vi "LSX Get Trigger Par.vi"(0 "lLSID":i32, 1 "pdDistance":dbl, 5 "plAxis":i32, 7 "plMode":i32, 9 "plSignal":i32, 11 "error in (no error)":errorcluster) -> (3 "pdDistance out":dbl, 4 "function return":i32, 6 "plAxis out":i32, 8 "plMode out":i32, 10 "plSignal out":i32, 15 "error out":errorcluster)   [LabVIEW 2018, in "Tango.lvlib"]
doc: "TANGOAPI int TANGOCALL LSX_GetTriggerPar (int lLSID, int *plAxis, int *plMode, int *plSignal, double *pdDistance);"
uses:
  Tango.lvlib
  SubVIs/Tango_DLL.dll
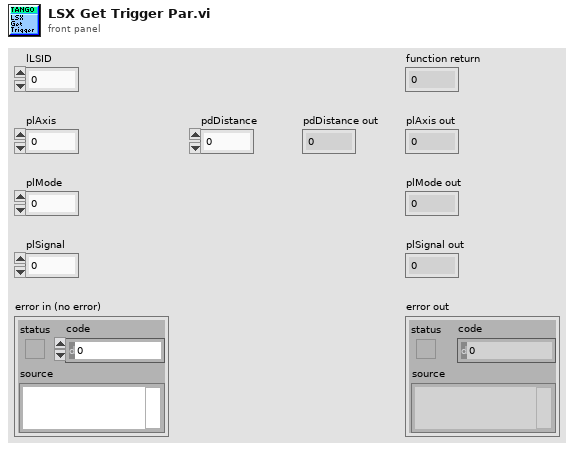
[diagram p1: front panel]
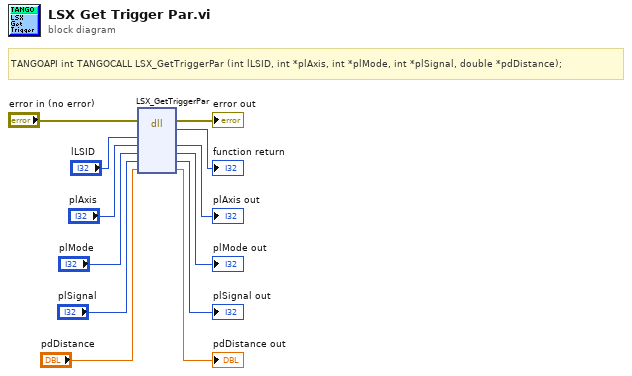
[diagram p0: block diagram]
diagram:
  # "TANGOAPI int TANGOCALL LSX_GetTriggerPar (int lLSID, int *plAxis, int *plMode, int *plSignal, double *pdDistance);"
  n1 = dll-call lib="C:/Users/Familie/Documents/LabviewIX81/lib/TANGO Stage/SubVIs/Tango_DLL.*" fn="LSX_GetTriggerPar"(error in="error in (no error)", "lLSID"="lLSID", "plAxis"="plAxis", "plMode"="plMode", "plSignal"="plSignal", "pdDistance"="pdDistance") -> (error out=→"error out":errorcluster, →"function return":i32, "plAxis"=→"plAxis out":i32, "plMode"=→"plMode out":i32, "plSignal"=→"plSignal out":i32, "pdDistance"=→"pdDistance out":dbl)  [unwired: 3 in, 1 out]
